vi "state cluster to channels.vi"(11 "state module configuration":T1) -> (3 "channels":refnum<class "TBM channel.lvclass">[](array[class]))   [LabVIEW 2013, in "user tag bus module configuration.lvclass"]
uses:
  user tag bus module configuration.lvclass
  <vilib>/NI/Tag Bus Module Framework/channel/TBM channel.lvclass
  state module configuration.ctl
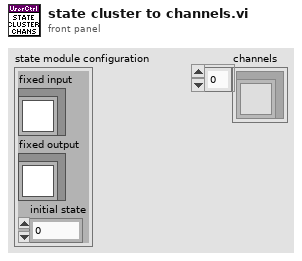
[diagram p1: front panel]
types:
  T1 = typedef "user tag bus module configuration.lvclass/state module configuration.ctl" = cluster{"fixed input":refnum<class "TBM channel.lvclass">, "fixed output":refnum<class "TBM channel.lvclass">, "initial state":u8}
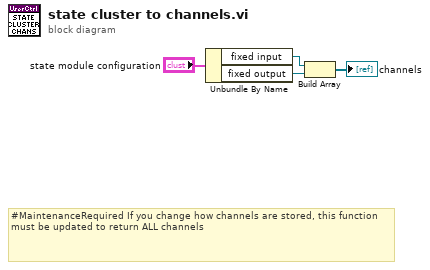
[diagram p0: block diagram]
diagram:
  # "#MaintenanceRequired If you change how channels are stored, this function must be updated to return ALL channels"
  n1 = Unbundle By Name("state module configuration") -> ("fixed input"=w2:refnum<class "TBM channel.lvclass">, "fixed output"=w4:refnum<class "TBM channel.lvclass">)
  n2 = Build Array(w2, w4) -> (→"channels":refnum<class "TBM channel.lvclass">[])
